vi "Sequence.Code.FirstSerial.vi"(0 "Serial in":i32, 1 "Code":T1={"LaserJob"="", "AdditionalTxt"="", "FactoryCode"="037", "RevID"=0, "ForkID"=0, "FailuresLimit"=0, "GlobalCnt"=0, "ScannerProgram"=0, "SerialFormat"=enum."6 dig", "CoordA"={"X"=0.0, "Y"=0.0, "Angle"=0.0}, "CoordB"={"X"=0.0, "Y"=0.0, "Angle"=0.0}, "DMCconfig"=0}, 2 "Printed serials":i32[](array[numeric])) -> (3 "Serial out":i32)   [LabVIEW 2016]
uses:
  Station/Station.Plate.Properties.ctl
  Sequence.Code.SerialFormat.ctl
  Drivers/V7310/LowLevel/V7310.Job.Sets.ctl
  Global/ApplicationGlobal.vi
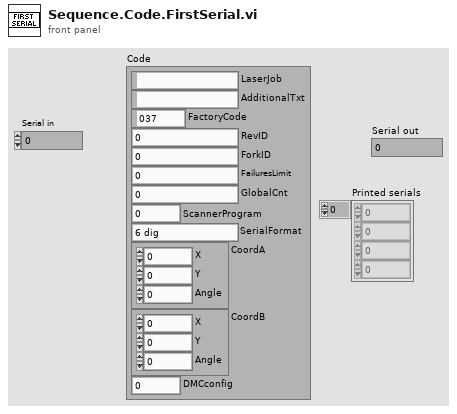
[diagram p1: front panel]
types:
  T1 = typedef "Station.Plate.Properties.ctl" = cluster{"LaserJob":string, "AdditionalTxt":string, "FactoryCode":string, "RevID":u8, "ForkID":u8, "FailuresLimit":u16, "GlobalCnt":i32, "ScannerProgram":u8, "SerialFormat":T2, "CoordA":T3, "CoordB":T3, "DMCconfig":i32}
  T2 = typedef "Sequence.Code.SerialFormat.ctl" = enum8{"", "6 dig", "7 dig"}
  T3 = typedef "V7310.Job.Sets.ctl" = cluster{"X":dbl, "Y":dbl, "Angle":dbl}
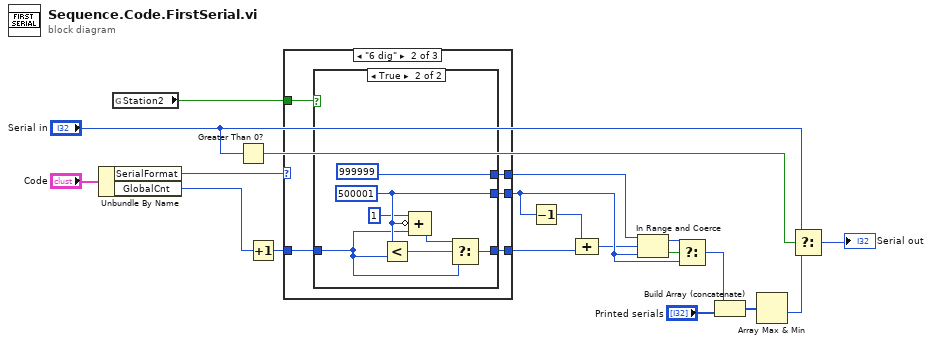
[diagram p0: block diagram]
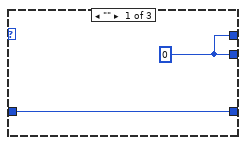
[diagram p2: hidden frame]
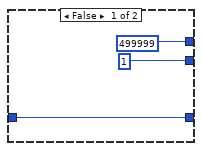
[diagram p3: hidden frame]
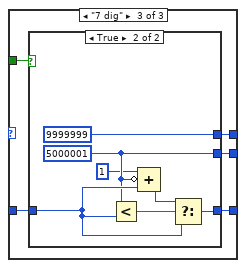
[diagram p4: hidden frame]
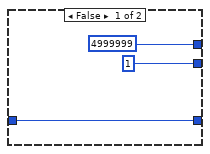
[diagram p5: hidden frame]
diagram:
  n1 = Unbundle By Name("Code") -> ("SerialFormat"=w16:T2, "GlobalCnt"=w3:i32)
  n2 = global read "ApplicationGlobal.vi" "Station2"() -> (w7:bool)
  n3 = Greater Than 0?(x="Serial in") -> (x > 0?=w9:bool)
  n4 = Increment(x=w3) -> (x+1=w10:i32)
  n5 = case shown="\"6 dig\"" w16 {
    tunnel: [w21 w25 w38] -> w14
    tunnel: [w21 w26 w41] -> w17
    tunnel: w10 -> [w20 w24 w39]
    tunnel: [w20 w23 w40] -> w11
    tunnel: w7 -> [_ w22 w37]
    frame "" {
      w21 = 0 ("Serial")
    }
    frame "6 dig" {
      n6 = case shown="True" w22 {
        tunnel: [499999 ("Serial") 999999 ("Serial")] -> w26
        tunnel: [1 ("Serial") w34] -> w25
        tunnel: w24 -> [w27 w32]
        tunnel: [w27 w31] -> w23
        frame False {
        }
        frame True {
          w34 = 500001 ("Serial")
          n7 = Less?(x=w34, y=w32) -> (x < y?=w35:bool)
          n8 = Compound Arithmetic op=ADD(1 ("value"), invert w34, w32) -> (w33:i32)
          n9 = Select(t=w33, s=w35, f=w32) -> (s? t:f=w31:i32)
        }
      }
    }
    frame "7 dig" {
      n10 = case shown="True" w37 {
        tunnel: [4999999 ("Serial") 9999999 ("Serial")] -> w41
        tunnel: [w42 w48] -> w40
        tunnel: w39 -> [w42 w47]
        tunnel: [1 ("Serial") w46] -> w38
        frame False {
        }
        frame True {
          w46 = 5000001 ("Serial")
          n11 = Less?(x=w46, y=w47) -> (x < y?=w50:bool)
          n12 = Compound Arithmetic op=ADD(1 ("value"), invert w46, w47) -> (w49:i32)
          n13 = Select(t=w49, s=w50, f=w47) -> (s? t:f=w48:i32)
        }
      }
    }
  }
  n14 = Decrement(x=w14) -> (x-1=w12:i32)
  n15 = Compound Arithmetic op=ADD(w12, w11) -> (w13:i32)
  n16 = In Range and Coerce(upper limit=w17, x=w13, lower limit=w14) -> (coerced(x)=w18:i32, In Range?=w19:bool)
  n17 = Select(t=w18, s=w19, f=w14) -> (s? t:f=w2:i32)
  n18 = Build Array (concatenate)(w2, "Printed serials") -> (w5:i32[])
  n19 = Array Max & Min(array=w5) -> (min value=w1:i32)  [unwired: 3 out]
  n20 = Select(t="Serial in", s=w9, f=w1) -> (s? t:f=→"Serial out":i32)
